vi "DBL GT 0.vi"(1 "DBL":dbl) -> (0 "DBL >= 0":dbl)   [LabVIEW 2011]
doc: "Coerces DBL value to >=0.\n\n\nVersion 1.0 - 02/13/2013\n\nPhaeron, Inc.\nwww.phaeron.com\ninfo@phaeron.com"
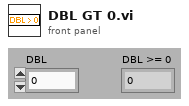
[diagram p1: front panel]
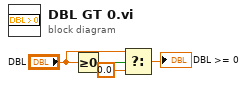
[diagram p0: block diagram]
diagram:
  n1 = Greater Or Equal To 0?(x="DBL") -> (x >= 0?=w3:bool)
  n2 = Select(t="DBL", s=w3, f=0.0) -> (s? t:f=→"DBL >= 0":dbl)
